vi "To Pretty String (Object).vi"(6 "pretty print? (T)":bool=TRUE, 7 "enable LabVIEW extensions? (T)":bool=TRUE, 8 "error in (no error)":errorcluster, 10 "indent":i32, 11 "JSON Value in":variant) -> (0 "error out":errorcluster, 3 "Pretty Print String":string)   [LabVIEW 2017, in "JSON Support for LabVIEW.lvlib"]
doc: "Pretty prints the given JSON data in an easier to read format."
uses:
  JSON Support for LabVIEW.lvlib
  Cluster Manipulation API.lvlib
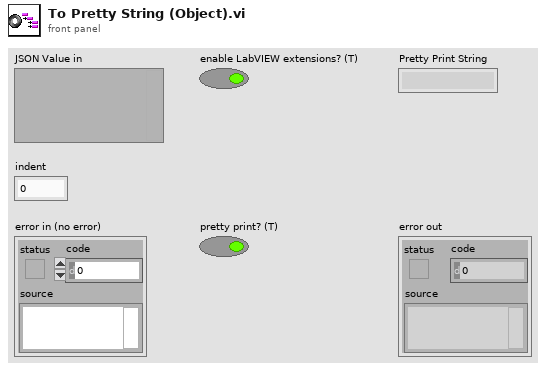
[diagram p1: front panel]
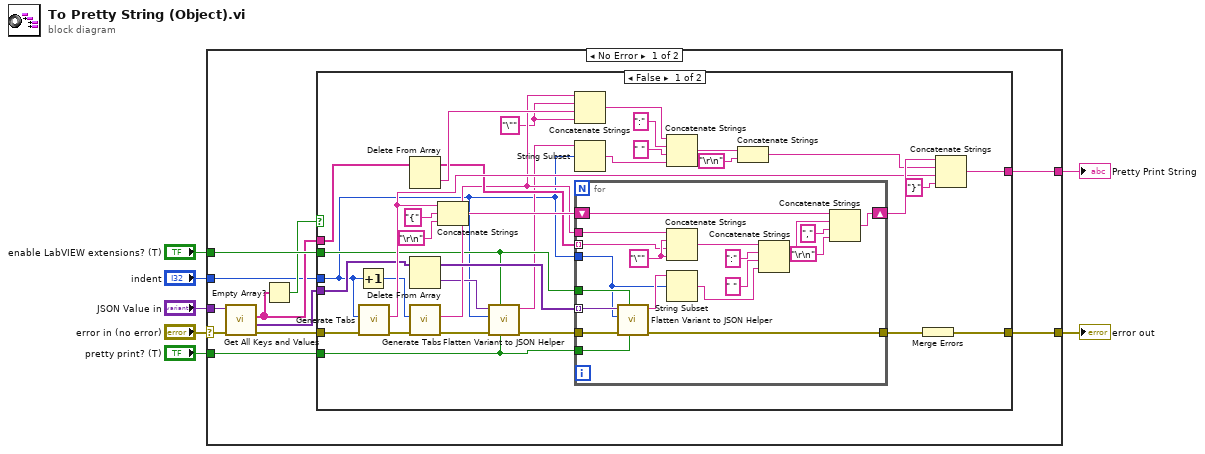
[diagram p0: block diagram]
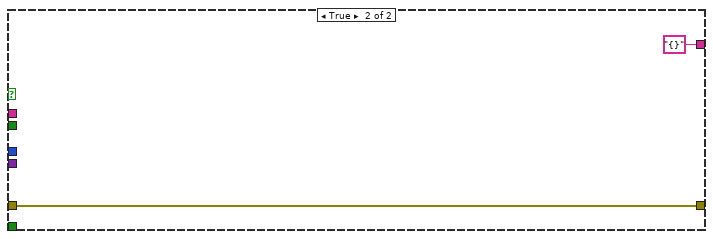
[diagram p2: hidden frame]
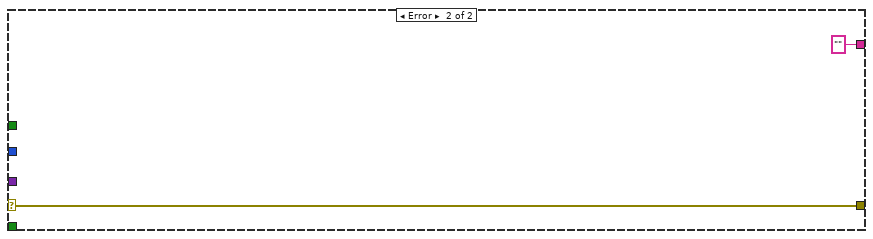
[diagram p3: hidden frame]
diagram:
  n1 = case shown="No Error" "error in (no error)" {
    selector: "error in (no error)" -> [w9 w73]
    tunnel: [w18 ""] -> w7
    tunnel: [w17 w73] -> w6
    tunnel: "JSON Value in" -> [w15 _]
    tunnel: "enable LabVIEW extensions? (T)" -> [w14 _]
    tunnel: "pretty print? (T)" -> [w13 _]
    tunnel: "indent" -> [w10 _]
    frame No Error {
      n2 = call "Get All Keys and Values.vi"("error in"=w9, "JSON Value in"=w15) -> ("error out"=w8:errorcluster, "values"=w16:variant[], "keys"=w11:string[])  [unwired: 7 in]
      n3 = Empty Array?(array=w11) -> (empty?=w12:bool)
      n4 = case shown="False" w12 {
        tunnel: [w42 "{}"] -> w18
        tunnel: [w49 w71] -> w17
        tunnel: w8 -> [w41 w71]
        tunnel: w16 -> [w40 _]
        tunnel: w14 -> [w32 _]
        tunnel: w13 -> [w31 _]
        tunnel: w11 -> [w30 _]
        tunnel: w10 -> [w19 _]
        frame False {
          w26 = "\"" ("string")
          n5 = Increment(x=w19) -> (x+1=w22:i32)
          n6 = call "Generate Tabs.vi"("error in (no error)"=w41, "indent"=w19) -> ("error out"=w29:errorcluster, "Tabs"=w43:string)  [unwired: 8 in]
          n7 = Delete From Array(array=w30) -> (deleted portion=w39:string, array with subset deleted=w38:string[])  [unwired: 2 in]
          n8 = Delete From Array(array=w40) -> (deleted portion=w35:variant, array with subset deleted=w48:variant[])  [unwired: 2 in]
          n9 = call "Generate Tabs.vi"("error in (no error)"=w29, "indent"=w22) -> ("error out"=w34:errorcluster, "Tabs"=w37:string)  [unwired: 8 in]
          n10 = Concatenate Strings(w43, "{" ("string"), "\r\n") -> (w50:string)
          n11 = call "Flatten Variant to JSON Helper.vi"("pretty print? (T)"=w31, "enable LabVIEW extensions? (T)"=w32, "error in (no error)"=w34, "indent"=w19, "JSON Value in"=w35) -> ("error out"=w33:errorcluster, "String"=w21:string)  [unwired: 5 in]
          n12 = Concatenate Strings(w37, w26, w39, w26) -> (w25:string)
          n13 = String Subset(string=w21, offset (0)=w19) -> (substring=w20:string)  [unwired: 1 in]
          n14 = for {
            tunnel: w48 -> [w58] mode=indexing
            shift-right: [w68] -> w47
            shift-left: w50 -> [w67]
            tunnel: w37 -> [w60]
            tunnel: w38 -> [w63] mode=indexing
            tunnel: w33 -> [w59]
            tunnel: [w57] -> w36
            tunnel: w32 -> [w56]
            tunnel: w31 -> [w55]
            tunnel: w19 -> [w52]
            w65 = "\"" ("string")
            n15 = call "Flatten Variant to JSON Helper.vi"("pretty print? (T)"=w55, "enable LabVIEW extensions? (T)"=w56, "error in (no error)"=w59, "indent"=w52, "JSON Value in"=w58) -> ("error out"=w57:errorcluster, "String"=w54:string)  [unwired: 5 in]
            n16 = Concatenate Strings(w60, w65, w63, w65) -> (w66:string)
            n17 = String Subset(string=w54, offset (0)=w52) -> (substring=w53:string)  [unwired: 1 in]
            n18 = Concatenate Strings(w66, ":" ("string"), " " ("string"), w53) -> (w62:string)
            n19 = Concatenate Strings(w67, w62, "," ("string"), "\r\n") -> (w68:string)
          }
          n20 = Concatenate Strings(w25, ":" ("string"), " " ("string"), w20) -> (w24:string)
          n21 = Concatenate Strings(w24, "\r\n") -> (w46:string)
          n22 = Merge Errors(w36) -> (w49:errorcluster)
          n23 = Concatenate Strings(w47, w46, w43, "}" ("string")) -> (w42:string)
        }
        frame True {
        }
      }
    }
    frame Error {
    }
  }
  "error out" <- w6
  "Pretty Print String" <- w7
